vi "wave-1.vi"(6 "offset signal":dbl=2.0, 7 "slope":dbl=0.1, 8 "N cycles":i64=3, 9 "Density":i64=100) -> (0 "signal":dbl[](graph)=[0.0, 0.0, 0.0, 0.0, 0.0, 0.0, 0.0, 0.0, 0.0, 0.0, 0.0, 0.0, 0.0, 0.0, 0.0, 0.0, 0.0, 0.0, 0.0, 0.0, 0.0, 0.0, 0.0, 0.0, 0.0, 0.0, 0.0, 0.0, 0.0, 0.0, 0.0, 0.0, 0.0, 0.0, 0.0, 0.0, 0.0, 0.0, 0.0, 0.0, 0.0, 0.0, 0.0, 0.0, 0.0, 0.0, 0.0, 0.0, 0.0, 0.0, 2.0, 2.001745328365898, 2.0034906567317967, 2.005235985097695, 2.0069813134635934, 2.0087266418294916, 2.0104719701953897, 2.0122172985612883, 2.0139626269271864, 2.015707955293085, 2.017453283658983, 2.0191986120248813, 2.02094394039078, 2.022689268756678, 2.024434597122576, 2.0261799254884747, 2.027925253854373, 2.0296705822202714, 2.0314159105861695, 2.0331612389520677, 2.0349065673179663, 2.0366518956838644, 2.038397224049763, 2.040142552415661, 2.0418878807815593, 2.043633209147458, 2.045378537513356, 2.0471238658792545, 2.0488691942451527, 2.050614522611051, 2.0523598509769494, 2.0541051793428475, 2.0558505077087457, 2.0575958360746442, 2.0593411644405424, 2.061086492806441, 2.062831821172339, 2.0645771495382372, 2.066322477904136, 2.068067806270034, 2.0698131346359325, 2.0715584630018307, 2.073303791367729, 2.0750491197336274, 2.0767944480995255, 2.078539776465424, 2.0802851048313222, 2.0820304331972204, 2.083775761563119, 2.085521089929017, 2.0872664182949157, 2.089011746660814, 2.090757075026712, 2.0925024033926105, 2.0942477317585086, 2.095993060124407, 2.0977383884903054, 2.0994837168562035, 2.101229045222102, 2.102974373588, 2.1047197019538983, 2.106465030319797, 2.108210358685695, 2.1099556870515936, 2.111701015417492, 2.11344634378339, 2.1151916721492885, 2.1169370005151866, 2.118682328881085, 2.1204276572469833, 2.1221729856128815, 2.12391831397878, 2.125663642344678, 2.1274089707105768, 2.129154299076475, 2.130899627442373, 2.1326449558082716, 2.1343902841741698, 2.136135612540068, 2.1378809409059665, 2.1396262692718646, 2.141371597637763, 2.1431169260036613, 2.1448622543695595, 2.146607582735458, 2.148352911101356, 2.1500982394672548, 2.151843567833153, 2.153588896199051, 2.1553342245649496, 2.1570795529308477, 2.158824881296746, 2.1605702096626445, 2.1623155380285426, 2.164060866394441, 2.1658061947603393, 2.1675515231262374, 2.169296851492136, 2.171042179858034, 2.1727875082239327, 0.0, 0.0, 0.0, 0.0, 0.0, 0.0, 0.0, 0.0, 0.0, 0.0, 0.0, 0.0, 0.0, 0.0, 0.0, 0.0, 0.0, 0.0, 0.0, 0.0, 0.0, 0.0, 0.0, 0.0, 0.0, 0.0, 0.0, 0.0, 0.0, 0.0, 0.0, 0.0, 0.0, 0.0, 0.0, 0.0, 0.0, 0.0, 0.0, 0.0, 0.0, 0.0, 0.0, 0.0, 0.0, 0.0, 0.0, 0.0, 0.0, 0.0, 0.0, 0.0, 0.0, 0.0, 0.0, 0.0, 0.0, 0.0, 0.0, 0.0, 0.0, 0.0, 0.0, 0.0, 0.0, 0.0, 0.0, 0.0, 0.0, 0.0, 0.0, 0.0, 0.0, 0.0, 0.0, 0.0, 0.0, 0.0, 0.0, 0.0, 0.0, 0.0, 0.0, 0.0, 0.0, 0.0, 0.0, 0.0, 0.0, 0.0, 0.0, 0.0, 0.0, 0.0, 0.0, 0.0, 0.0, 0.0, 0.0, 0.0, 2.0, 2.001745328365898, 2.0034906567317967, 2.005235985097695, 2.0069813134635934, 2.0087266418294916, 2.0104719701953897, 2.0122172985612883, 2.0139626269271864, 2.015707955293085, 2.017453283658983, 2.0191986120248813, 2.02094394039078, 2.022689268756678, 2.024434597122576, 2.0261799254884747, 2.027925253854373, 2.0296705822202714, 2.0314159105861695, 2.0331612389520677, 2.0349065673179663, 2.0366518956838644, 2.038397224049763, 2.040142552415661, 2.0418878807815593, 2.043633209147458, 2.045378537513356, 2.0471238658792545, 2.0488691942451527, 2.050614522611051, 2.0523598509769494, 2.0541051793428475, 2.0558505077087457, 2.0575958360746442, 2.0593411644405424, 2.061086492806441, 2.062831821172339, 2.0645771495382372, 2.066322477904136, 2.068067806270034, 2.0698131346359325, 2.0715584630018307, 2.073303791367729, 2.0750491197336274, 2.0767944480995255, 2.078539776465424, 2.0802851048313222, 2.0820304331972204, 2.083775761563119, 2.085521089929017, 2.0872664182949157, 2.089011746660814, 2.090757075026712, 2.0925024033926105, 2.0942477317585086, 2.095993060124407, 2.0977383884903054, 2.0994837168562035, 2.101229045222102, 2.102974373588, 2.1047197019538983, 2.106465030319797, 2.108210358685695, 2.1099556870515936, 2.111701015417492, 2.11344634378339, 2.1151916721492885, 2.1169370005151866, 2.118682328881085, 2.1204276572469833, 2.1221729856128815, 2.12391831397878, 2.125663642344678, 2.1274089707105768, 2.129154299076475, 2.130899627442373, 2.1326449558082716, 2.1343902841741698, 2.136135612540068, 2.1378809409059665, 2.1396262692718646, 2.141371597637763, 2.1431169260036613, 2.1448622543695595, 2.146607582735458, 2.148352911101356, 2.1500982394672548, 2.151843567833153, 2.153588896199051, 2.1553342245649496, 2.1570795529308477, 2.158824881296746, 2.1605702096626445, 2.1623155380285426, 2.164060866394441, 2.1658061947603393, 2.1675515231262374, 2.169296851492136, 2.171042179858034, 2.1727875082239327, 0.0, 0.0, 0.0, 0.0, 0.0, 0.0, 0.0, 0.0, 0.0, 0.0, 0.0, 0.0, 0.0, 0.0, 0.0, 0.0, 0.0, 0.0, 0.0, 0.0, 0.0, 0.0, 0.0, 0.0, 0.0, 0.0, 0.0, 0.0, 0.0, 0.0, 0.0, 0.0, 0.0, 0.0, 0.0, 0.0, 0.0, 0.0, 0.0, 0.0, 0.0, 0.0, 0.0, 0.0, 0.0, 0.0, 0.0, 0.0, 0.0, 0.0, 0.0, 0.0, 0.0, 0.0, 0.0, 0.0, 0.0, 0.0, 0.0, 0.0, 0.0, 0.0, 0.0, 0.0, 0.0, 0.0, 0.0, 0.0, 0.0, 0.0, 0.0, 0.0, 0.0, 0.0, 0.0, 0.0, 0.0, 0.0, 0.0, 0.0, 0.0, 0.0, 0.0, 0.0, 0.0, 0.0, 0.0, 0.0, 0.0, 0.0, 0.0, 0.0, 0.0, 0.0, 0.0, 0.0, 0.0, 0.0, 0.0, 0.0, 2.0, 2.001745328365898, 2.0034906567317967, 2.005235985097695, 2.0069813134635934, 2.0087266418294916, 2.0104719701953897, 2.0122172985612883, 2.0139626269271864, 2.015707955293085, 2.017453283658983, 2.0191986120248813, 2.02094394039078, 2.022689268756678, 2.024434597122576, 2.0261799254884747, 2.027925253854373, 2.0296705822202714, 2.0314159105861695, 2.0331612389520677, 2.0349065673179663, 2.0366518956838644, 2.038397224049763, 2.040142552415661, 2.0418878807815593, 2.043633209147458, 2.045378537513356, 2.0471238658792545, 2.0488691942451527, 2.050614522611051, 2.0523598509769494, 2.0541051793428475, 2.0558505077087457, 2.0575958360746442, 2.0593411644405424, 2.061086492806441, 2.062831821172339, 2.0645771495382372, 2.066322477904136, 2.068067806270034, 2.0698131346359325, 2.0715584630018307, 2.073303791367729, 2.0750491197336274, 2.0767944480995255, 2.078539776465424, 2.0802851048313222, 2.0820304331972204, 2.083775761563119, 2.085521089929017, 2.0872664182949157, 2.089011746660814, 2.090757075026712, 2.0925024033926105, 2.0942477317585086, 2.095993060124407, 2.0977383884903054, 2.0994837168562035, 2.101229045222102, 2.102974373588, 2.1047197019538983, 2.106465030319797, 2.108210358685695, 2.1099556870515936, 2.111701015417492, 2.11344634378339, 2.1151916721492885, 2.1169370005151866, 2.118682328881085, 2.1204276572469833, 2.1221729856128815, 2.12391831397878, 2.125663642344678, 2.1274089707105768, 2.129154299076475, 2.130899627442373, 2.1326449558082716, 2.1343902841741698, 2.136135612540068, 2.1378809409059665, 2.1396262692718646, 2.141371597637763, 2.1431169260036613, 2.1448622543695595, 2.146607582735458, 2.148352911101356, 2.1500982394672548, 2.151843567833153, 2.153588896199051, 2.1553342245649496, 2.1570795529308477, 2.158824881296746, 2.1605702096626445, 2.1623155380285426, 2.164060866394441, 2.1658061947603393, 2.1675515231262374, 2.169296851492136, 2.171042179858034, 2.1727875082239327, 0.0, 0.0, 0.0, 0.0, 0.0, 0.0, 0.0, 0.0, 0.0, 0.0, 0.0, 0.0, 0.0, 0.0, 0.0, 0.0, 0.0, 0.0, 0.0, 0.0, 0.0, 0.0, 0.0, 0.0, 0.0, 0.0, 0.0, 0.0, 0.0, 0.0, 0.0, 0.0, 0.0, 0.0, 0.0, 0.0, 0.0, 0.0, 0.0, 0.0, 0.0, 0.0, 0.0, 0.0, 0.0, 0.0, 0.0, 0.0, 0.0, 0.0], 3 "trigger":i32[](graph)=[5, 5, 5, 5, 5, 5, 5, 5, 5, 5, 5, 5, 5, 5, 5, 5, 5, 5, 5, 5, 5, 5, 5, 5, 5, 5, 5, 5, 5, 5, 5, 5, 5, 5, 5, 5, 5, 5, 5, 5, 5, 5, 5, 5, 5, 5, 5, 5, 5, 5, 5, 5, 5, 5, 5, 5, 5, 5, 5, 5, 5, 5, 5, 5, 5, 5, 5, 5, 5, 5, 5, 5, 5, 5, 5, 5, 5, 5, 5, 5, 5, 5, 5, 5, 5, 5, 5, 5, 5, 5, 5, 5, 5, 5, 5, 5, 5, 5, 5, 5, 0, 0, 0, 0, 0, 0, 0, 0, 0, 0, 0, 0, 0, 0, 0, 0, 0, 0, 0, 0, 0, 0, 0, 0, 0, 0, 0, 0, 0, 0, 0, 0, 0, 0, 0, 0, 0, 0, 0, 0, 0, 0, 0, 0, 0, 0, 0, 0, 0, 0, 0, 0, 0, 0, 0, 0, 0, 0, 0, 0, 0, 0, 0, 0, 0, 0, 0, 0, 0, 0, 0, 0, 0, 0, 0, 0, 0, 0, 0, 0, 0, 0, 0, 0, 0, 0, 0, 0, 0, 0, 0, 0, 0, 0, 0, 0, 0, 0, 0, 0, 5, 5, 5, 5, 5, 5, 5, 5, 5, 5, 5, 5, 5, 5, 5, 5, 5, 5, 5, 5, 5, 5, 5, 5, 5, 5, 5, 5, 5, 5, 5, 5, 5, 5, 5, 5, 5, 5, 5, 5, 5, 5, 5, 5, 5, 5, 5, 5, 5, 5, 5, 5, 5, 5, 5, 5, 5, 5, 5, 5, 5, 5, 5, 5, 5, 5, 5, 5, 5, 5, 5, 5, 5, 5, 5, 5, 5, 5, 5, 5, 5, 5, 5, 5, 5, 5, 5, 5, 5, 5, 5, 5, 5, 5, 5, 5, 5, 5, 5, 5, 0, 0, 0, 0, 0, 0, 0, 0, 0, 0, 0, 0, 0, 0, 0, 0, 0, 0, 0, 0, 0, 0, 0, 0, 0, 0, 0, 0, 0, 0, 0, 0, 0, 0, 0, 0, 0, 0, 0, 0, 0, 0, 0, 0, 0, 0, 0, 0, 0, 0, 0, 0, 0, 0, 0, 0, 0, 0, 0, 0, 0, 0, 0, 0, 0, 0, 0, 0, 0, 0, 0, 0, 0, 0, 0, 0, 0, 0, 0, 0, 0, 0, 0, 0, 0, 0, 0, 0, 0, 0, 0, 0, 0, 0, 0, 0, 0, 0, 0, 0, 5, 5, 5, 5, 5, 5, 5, 5, 5, 5, 5, 5, 5, 5, 5, 5, 5, 5, 5, 5, 5, 5, 5, 5, 5, 5, 5, 5, 5, 5, 5, 5, 5, 5, 5, 5, 5, 5, 5, 5, 5, 5, 5, 5, 5, 5, 5, 5, 5, 5, 5, 5, 5, 5, 5, 5, 5, 5, 5, 5, 5, 5, 5, 5, 5, 5, 5, 5, 5, 5, 5, 5, 5, 5, 5, 5, 5, 5, 5, 5, 5, 5, 5, 5, 5, 5, 5, 5, 5, 5, 5, 5, 5, 5, 5, 5, 5, 5, 5, 5, 0, 0, 0, 0, 0, 0, 0, 0, 0, 0, 0, 0, 0, 0, 0, 0, 0, 0, 0, 0, 0, 0, 0, 0, 0, 0, 0, 0, 0, 0, 0, 0, 0, 0, 0, 0, 0, 0, 0, 0, 0, 0, 0, 0, 0, 0, 0, 0, 0, 0, 0, 0, 0, 0, 0, 0, 0, 0, 0, 0, 0, 0, 0, 0, 0, 0, 0, 0, 0, 0, 0, 0, 0, 0, 0, 0, 0, 0, 0, 0, 0, 0, 0, 0, 0, 0, 0, 0, 0, 0, 0, 0, 0, 0, 0, 0, 0, 0, 0, 0])   [LabVIEW 2014]
doc: "André Romero - 2016\nandretec@ifsc.usp.br"
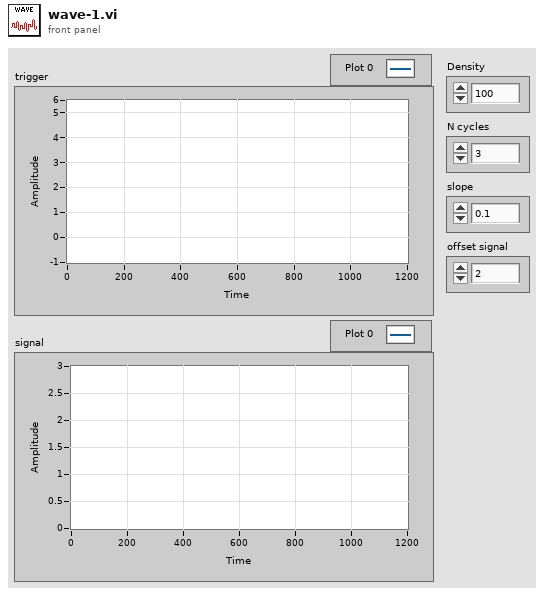
[diagram p1: front panel]
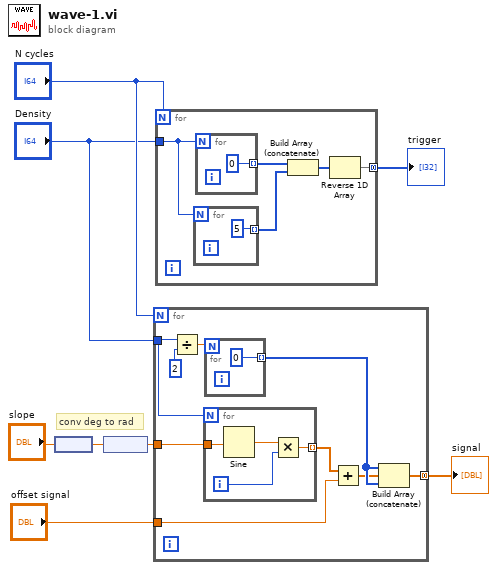
[diagram p0: block diagram]
diagram:
  # "conv deg to rad"
  n1 = node("slope") -> (w4:dbl[unit])
  n2 = node(w4) -> (w3:dbl)
  n3 = for {
    N: "N cycles" -> [_]
    tunnel: [w14] -> w6 mode=concatenating
    tunnel: "Density" -> [w13]
    tunnel: w3 -> [w12]
    tunnel: "offset signal" -> [w10]
    n4 = Divide(x=w13, y=2) -> (x/y=w17:dbl)
    n5 = for {
      N: w13 -> [_]
      tunnel: [w19] -> w11 mode=indexing
      tunnel: w12 -> [w18]
      i -> [w20]
      n6 = Sine(x=w18) -> (sin(x)=w21:dbl)
      n7 = Multiply(x=w21, y=w20) -> (x*y=w19:dbl)
    }
    n8 = for {
      N: w17 -> [_]
      tunnel: [0] -> w15 mode=indexing
    }
    n9 = Add(x=w11, y=w10) -> (x+y=w9:dbl[])
    n10 = Build Array (concatenate)(w15, w9, w15) -> (w14:dbl[])
  }
  "signal" <- w6
  n11 = for {
    N: "N cycles" -> [_]
    tunnel: [w24] -> w8 mode=concatenating
    tunnel: "Density" -> [w23]
    n12 = for {
      N: w23 -> [_]
      tunnel: [5] -> w26 mode=indexing
    }
    n13 = for {
      N: w23 -> [_]
      tunnel: [0] -> w27 mode=indexing
    }
    n14 = Build Array (concatenate)(w27, w26) -> (w25:i32[])
    n15 = Reverse 1D Array(array=w25) -> (reversed array=w24:i32[])
  }
  "trigger" <- w8
